vi "PhotonVision_ReadTargetData.vi"() -> ()   [LabVIEW 2019]
uses:
  <vilib>/Rock Robotics/WPI/ThirdParty/PhotonVisionLib/TypeDef/PhotonPipelineResultType.ctl
  <vilib>/Rock Robotics/WPI/ThirdParty/PhotonVisionLib/TypeDef/PhotonTrackedTargetType.ctl
  <vilib>/Rock Robotics/WPI/ThirdParty/PhotonVisionLib/TypeDef/TargetCornerType.ctl
  <vilib>/Rock Robotics/WPI/ThirdParty/JAS_Junk/TrajLib/TypeDef/TRANSFORM3D.ctl
  <vilib>/Rock Robotics/WPI/ThirdParty/JAS_Junk/TrajLib/TypeDef/TRANSLATION3D.ctl
  <vilib>/Rock Robotics/WPI/ThirdParty/JAS_Junk/TrajLib/TypeDef/ROTATION3D.ctl
  <vilib>/Rock Robotics/WPI/ThirdParty/JAS_Junk/TrajLib/TypeDef/QUATERNION.ctl
  <vilib>/Rock Robotics/WPI/ThirdParty/PhotonVisionLib/TypeDef/PhotonMultiTargetPNPResultType.ctl
  <vilib>/Rock Robotics/WPI/ThirdParty/PhotonVisionLib/TypeDef/PhotonPNPResultType.ctl
  <vilib>/Rock Robotics/WPI/ThirdParty/PhotonVisionLib/TypeDef/PhotonPipelineMetadataType.ctl
  <vilib>/Rock Robotics/WPI/ThirdParty/PhotonVisionLib/SubVI/PhotonPipelineResult_Unpack.vi
  <vilib>/Rock Robotics/WPI/ThirdParty/PhotonVisionLib/SubVI/PhotonPipelineResult_GetTargetCount.vi
  <vilib>/Rock Robotics/WPI/ThirdParty/PhotonVisionLib/SubVI/PhotonPipelineResult_GetMetadata.vi
  <vilib>/Rock Robotics/WPI/ThirdParty/PhotonVisionLib/SubVI/PhotonPipelineMetadata_GetAll.vi
  <vilib>/Rock Robotics/WPI/ThirdParty/PhotonVisionLib/SubVI/Packet_decode_ByteI8.vi
  <vilib>/Rock Robotics/WPI/ThirdParty/PhotonVisionLib/SubVI/PhotonTrackedTarget_Unpack.vi
  <vilib>/Rock Robotics/WPI/ThirdParty/PhotonVisionLib/SubVI/PhotonMultiTargetPNPResult_unpack.vi
  <vilib>/Rock Robotics/WPI/ThirdParty/PhotonVisionLib/SubVI/PhotonPipelineMetadata_Unpack.vi
  <vilib>/Rock Robotics/WPI/ThirdParty/PhotonVisionLib/SubVI/PhotonPipelineResult_New.vi
  <vilib>/Rock Robotics/WPI/ThirdParty/PhotonVisionLib/SubVI/Packet_decode_Flt64.vi
  <vilib>/Rock Robotics/WPI/ThirdParty/PhotonVisionLib/SubVI/TargetCorner_New.vi
  <vilib>/Rock Robotics/WPI/ThirdParty/PhotonVisionLib/SubVI/Packet_decode_Int32.vi
  <vilib>/Rock Robotics/WPI/ThirdParty/PhotonVisionLib/SubVI/Packet_decode_Transform3d.vi
  <vilib>/Rock Robotics/WPI/ThirdParty/PhotonVisionLib/SubVI/Packet_decode_Flt32.vi
  <vilib>/Rock Robotics/WPI/ThirdParty/PhotonVisionLib/SubVI/Packet_decode_TargetCornerArray.vi
  <vilib>/Rock Robotics/WPI/ThirdParty/PhotonVisionLib/SubVI/Packet_decode_Boolean.vi
  <vilib>/Rock Robotics/WPI/ThirdParty/PhotonVisionLib/SubVI/PhotonPNPResult_unpack.vi
  <vilib>/Rock Robotics/WPI/ThirdParty/PhotonVisionLib/SubVI/PhotonMultiTargetPNPResult_New.vi
  <vilib>/Rock Robotics/WPI/ThirdParty/PhotonVisionLib/SubVI/Packet_decode_Int16.vi
  <vilib>/Rock Robotics/WPI/ThirdParty/PhotonVisionLib/SubVI/Packet_decode_Int64.vi
  <vilib>/Rock Robotics/WPI/ThirdParty/JAS_Junk/TrajLib/VI/Transform3d_Create_Trans3dRot3d.vi
  <vilib>/Rock Robotics/WPI/ThirdParty/JAS_Junk/TrajLib/VI/Translation3d_Create.vi
  <vilib>/Rock Robotics/WPI/ThirdParty/JAS_Junk/TrajLib/VI/Rotation3d_Create_Quaternion.vi
  <vilib>/Rock Robotics/WPI/ThirdParty/JAS_Junk/TrajLib/VI/Quaternion_New.vi
  <vilib>/Rock Robotics/WPI/ThirdParty/PhotonVisionLib/SubVI/PhotonPNPResult_New.vi
  <vilib>/Rock Robotics/WPI/ThirdParty/JAS_Junk/TrajLib/VI/Quaternion_Normalize.vi
  <vilib>/Rock Robotics/WPI/ThirdParty/JAS_Junk/TrajLib/VI/Quaternion_New_Default.vi
  <vilib>/Rock Robotics/Network Tables/NT Write Boolean.vi
  <vilib>/Rock Robotics/Network Tables/NT Read Value.vi
  <vilib>/Rock Robotics/Network Tables/NT Read Raw.vi
  <vilib>/Rock Robotics/Network Tables/NT Write Number.vi
  <vilib>/Rock Robotics/WPI/ThirdParty/PhotonVisionLib/PhotonVisionLib.lvlib
  <vilib>/Rock Robotics/WPI/ThirdParty/JAS_Junk/TrajLib/Trajectory_Library.lvlib
panel:
  out "New Data":bool
  out "IsConnected":bool
  out "Has Targets":bool
  in  "CameraName":string="Microsoft LifeCam HD-3000"
  out "CtrlLibDistToBestTarg\nMeters":dbl
  out "Loop Count":i32
  out "SpecificPhotonTrackedTarget":T1={"Yaw"=0.0, "Pitch"=0.0, "Area"=0.0, "Skew"=0.0, "MinAreaRectCorners"=[], "BestCameraToTarget"={"TRANSLATION3D"={"X"=0.0, "Y"=0.0, "Z"=0.0}, "ROTATION3D"={"Q_quaternion"={"R"=1.0, "V"=[0.0, 0.0, 0.0]}}, "XF"=FALSE}, "FiducialId"=0, "AltCameraToTarget"={"TRANSLATION3D"={"X"=0.0, "Y"=0.0, "Z"=0.0}, "ROTATION3D"={"Q_quaternion"={"R"=0.0, "V"=[0.0, 0.0, 0.0]}}, "XF"=FALSE}, "PoseAmbiguity"=0.0, "DetectedCorners"=[], "ObjDetectId"=0, "ObjDetectConf"=0.0} {"AltCameraToTarget"."TRANSLATION3D"."Z" format="%14.3f"; "AltCameraToTarget"."TRANSLATION3D"."Y" format="%14.3f"; "AltCameraToTarget"."TRANSLATION3D"."X" format="%14.3f"; "BestCameraToTarget"."TRANSLATION3D"."Z" format="%14.3f"; "BestCameraToTarget"."TRANSLATION3D"."Y" format="%14.3f"; "BestCameraToTarget"."TRANSLATION3D"."X" format="%14.3f"}
  out "PipelineResult":T7={"Targets"=[], "PhotonMultiTargetPNPResult"={"PhotonPNPResult"={"IsPresent"=FALSE, "bestReprojErr"=0.0, "altReprojErr"=0.0, "ambiguity"=0.0, "Best"={"TRANSLATION3D"={"X"=0.0, "Y"=0.0, "Z"=0.0}, "ROTATION3D"={"Q_quaternion"={"R"=1.0, "V"=[0.0, 0.0, 0.0]}}, "XF"=FALSE}, "Alt"={"TRANSLATION3D"={"X"=0.0, "Y"=0.0, "Z"=0.0}, "ROTATION3D"={"Q_quaternion"={"R"=1.0, "V"=[0.0, 0.0, 0.0]}}, "XF"=FALSE}}, "FiducialIDsUsed"=[]}, "PhotonPipelineMetadata"={"CaptureTimestampMicros"=0, "PublishTimestampMicros"=0, "SequenceID"=0, "TimeSinceLastPong"=0}} {"PhotonMultiTargetPNPResult"."PhotonPNPResult"."Alt"."TRANSLATION3D"."Z" format="%14.3f"; "PhotonMultiTargetPNPResult"."PhotonPNPResult"."Alt"."TRANSLATION3D"."Y" format="%14.3f"; "PhotonMultiTargetPNPResult"."PhotonPNPResult"."Alt"."TRANSLATION3D"."X" format="%14.3f"; "PhotonMultiTargetPNPResult"."PhotonPNPResult"."Best"."TRANSLATION3D"."Z" format="%14.3f"; "PhotonMultiTargetPNPResult"."PhotonPNPResult"."Best"."TRANSLATION3D"."Y" format="%14.3f"; "PhotonMultiTargetPNPResult"."PhotonPNPResult"."Best"."TRANSLATION3D"."X" format="%14.3f"; "Targets"."AltCameraToTarget"."TRANSLATION3D"."Z" format="%14.3f"; "Targets"."AltCameraToTarget"."TRANSLATION3D"."Y" format="%14.3f"; "Targets"."AltCameraToTarget"."TRANSLATION3D"."X" format="%14.3f"; "Targets"."BestCameraToTarget"."TRANSLATION3D"."Z" format="%14.3f"; "Targets"."BestCameraToTarget"."TRANSLATION3D"."Y" format="%14.3f"; "Targets"."BestCameraToTarget"."TRANSLATION3D"."X" format="%14.3f"}
  out "SpecificTargetFound":bool
  out "TagTarget Index":i32
  in  "Fiiducial ID\n(April Tag Number)":i32
  out "BestTargetFound":bool
  out "BestYaw":dbl
  out "DistanceToBestTarget \nMeters":dbl
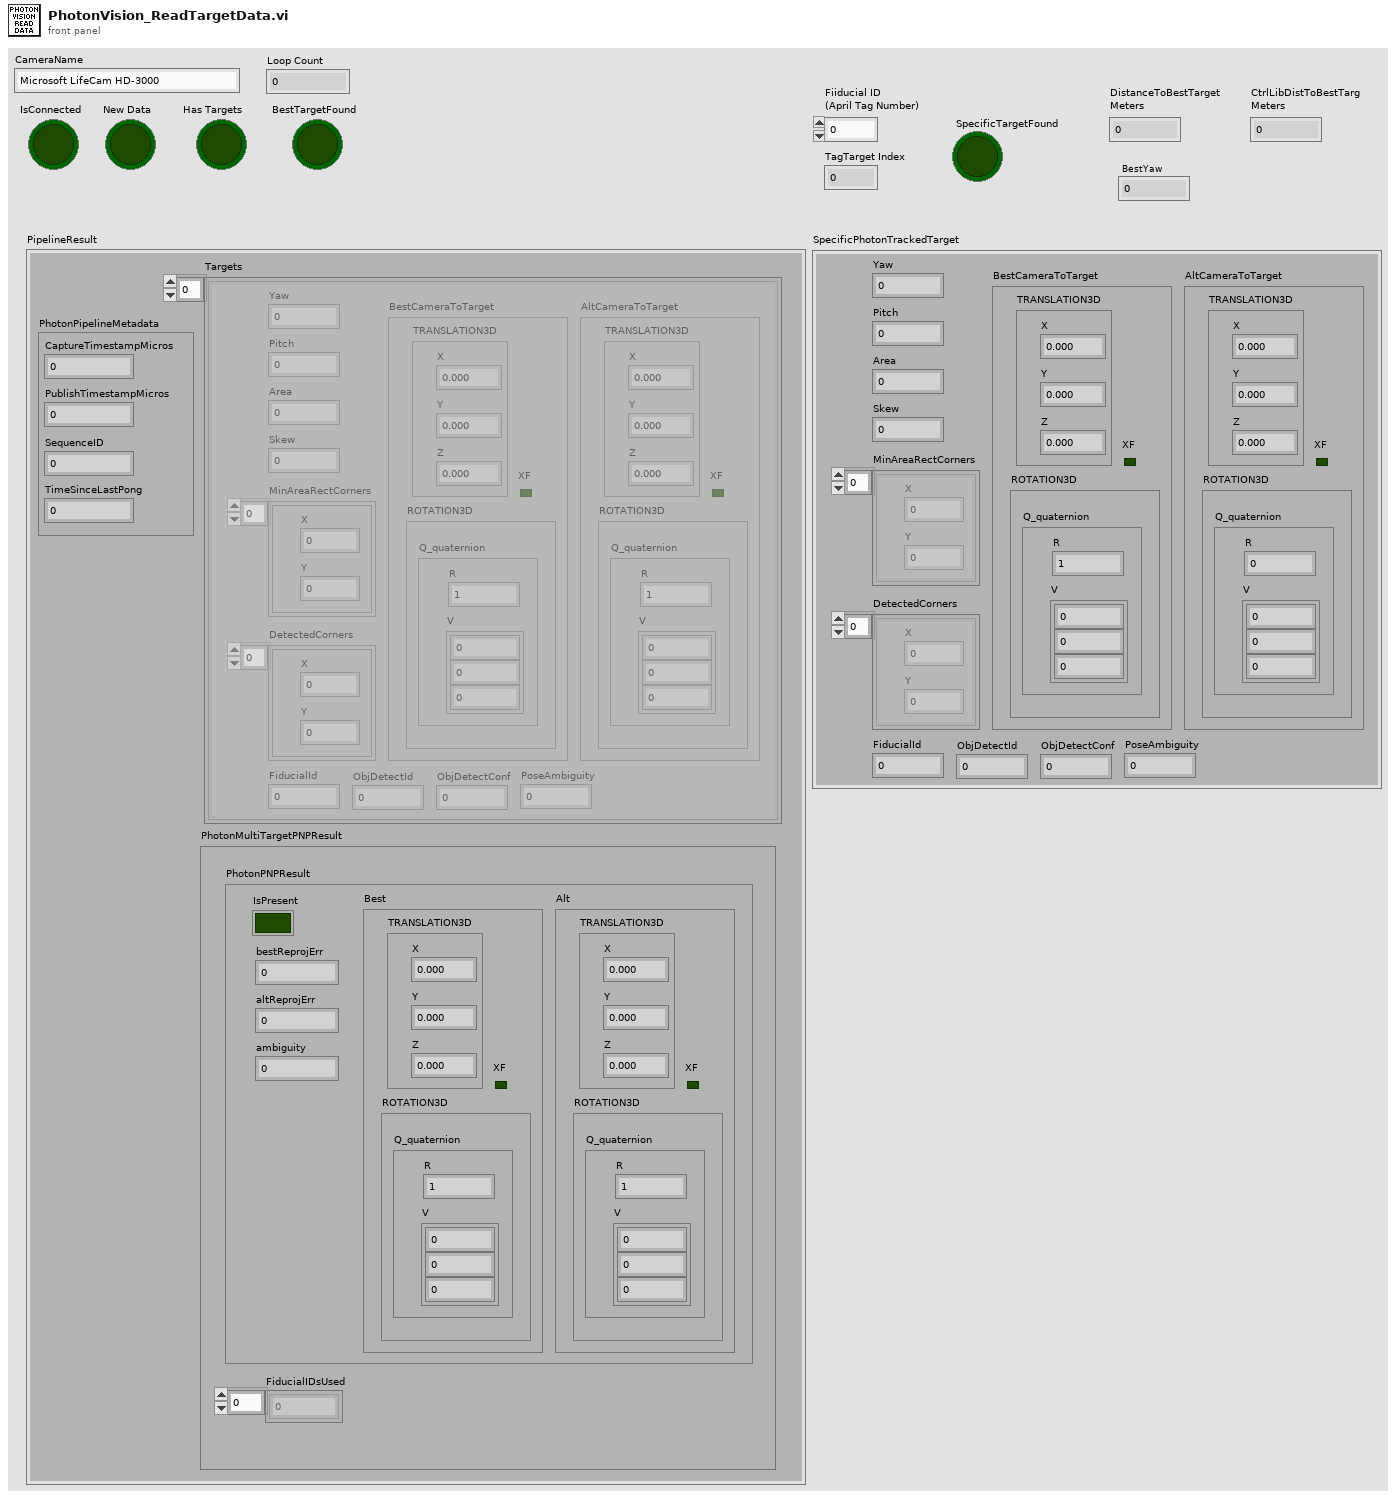
[diagram p1: front panel]
types:
  T1 = typedef "PhotonVisionLib.lvlib/PhotonTrackedTargetType.ctl" = cluster{"Yaw":dbl, "Pitch":dbl, "Area":dbl, "Skew":dbl, "MinAreaRectCorners":T2[], "BestCameraToTarget":T3, "FiducialId":i32, "AltCameraToTarget":T3, "PoseAmbiguity":dbl, "DetectedCorners":T2[], "ObjDetectId":i32, "ObjDetectConf":sgl}
  T2 = typedef "PhotonVisionLib.lvlib/TargetCornerType.ctl" = cluster{"X":dbl, "Y":dbl}
  T3 = typedef "Trajectory_Library.lvlib/TRANSFORM3D.ctl" = cluster{"TRANSLATION3D":T4, "ROTATION3D":T5, "XF":bool}
  T4 = typedef "Trajectory_Library.lvlib/TRANSLATION3D.ctl" = cluster{"X":dbl, "Y":dbl, "Z":dbl}
  T5 = typedef "Trajectory_Library.lvlib/ROTATION3D.ctl" = cluster{"Q_quaternion":T6}
  T6 = typedef "Trajectory_Library.lvlib/QUATERNION.ctl" = cluster{"R":dbl, "V":dbl[]}
  T7 = typedef "PhotonVisionLib.lvlib/PhotonPipelineResultType.ctl" = cluster{"Targets":T1[], "PhotonMultiTargetPNPResult":T8, "PhotonPipelineMetadata":T10}
  T8 = typedef "PhotonVisionLib.lvlib/PhotonMultiTargetPNPResultType.ctl" = cluster{"PhotonPNPResult":T9, "FiducialIDsUsed":i16[]}
  T9 = typedef "PhotonVisionLib.lvlib/PhotonPNPResultType.ctl" = cluster{"IsPresent":bool, "bestReprojErr":dbl, "altReprojErr":dbl, "ambiguity":dbl, "Best":T3, "Alt":T3}
  T10 = typedef "PhotonVisionLib.lvlib/PhotonPipelineMetadataType.ctl" = cluster{"CaptureTimestampMicros":i64, "PublishTimestampMicros":i64, "SequenceID":i64, "TimeSinceLastPong":i64}
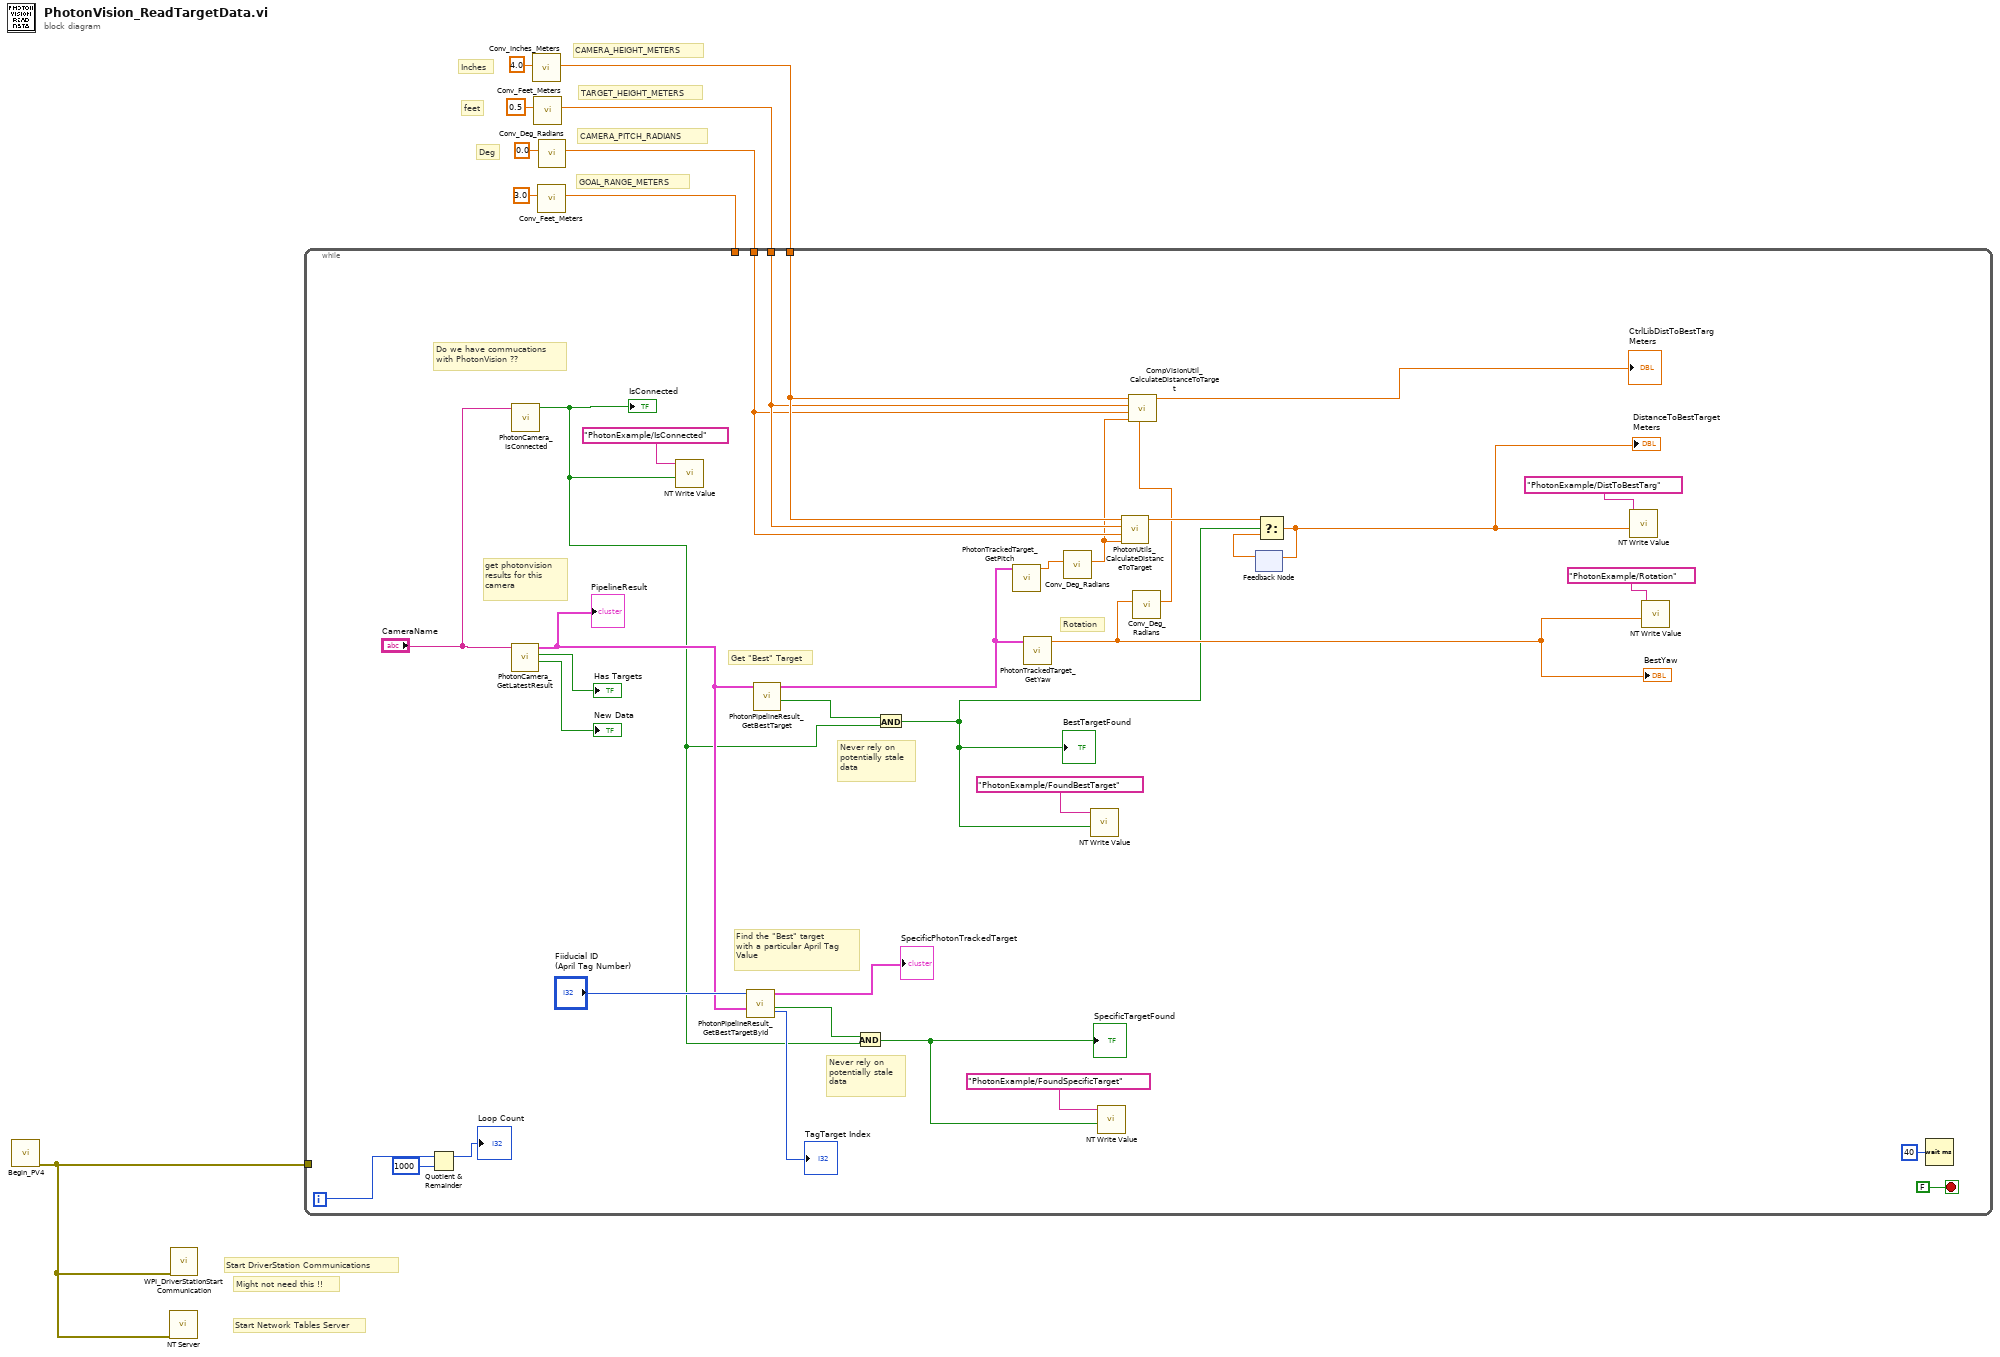
[diagram p0: block diagram]
diagram:
  # "Might not need this !!"
  # "Deg"
  # "feet"
  # "Inches"
  # "GOAL_RANGE_METERS"
  # "CAMERA_PITCH_RADIANS"
  # "TARGET_HEIGHT_METERS"
  # "CAMERA_HEIGHT_METERS"
  # "Start Network Tables Server"
  # "Start DriverStation Communications"
  n1 = call "Begin_PV4.vi"() -> ("error out"=w1:errorcluster)  [unwired: 11 in]
  n2 = call <vilib>:"NT Server.vi"("error in (no error)"=w1) -> ()  [unwired: 10 in, 1 out]
  n3 = call <vilib>:"WPI_DriverStationStart Communication.vi"("error in (no error)"=w1) -> ()  [unwired: 11 in]
  n4 = call <vilib>:"Conv_Inches_Meters.vi"("INCH"=4.0) -> ("Meters"=w5:dbl)  [unwired: 10 in]
  n5 = call <vilib>:"Conv_Feet_Meters.vi"("Feet"=0.5) -> ("Meters"=w4:dbl)  [unwired: 10 in]
  n6 = call <vilib>:"Conv_Feet_Meters.vi"("Feet"=3.0) -> ("Meters"=w2:dbl)  [unwired: 10 in]
  n7 = call <vilib>:"Conv_Deg_Radians.vi"("Degress"=0.0) -> ("Radians"=w3:dbl)  [unwired: 10 in]
  n8 = while {
    tunnel: w5 -> [w25]
    tunnel: w4 -> [w24]
    tunnel: w3 -> [w23]
    tunnel: w2 -> [_]
    tunnel: w1 -> [_]
    i -> [w28]
    stop <- FALSE stop-if-true
    # "Never rely on\npotentially stale\ndata"
    # "Never rely on\npotentially stale\ndata"
    # "Do we have commucations\nwith PhotonVision ??"
    # "Find the \"Best\" target\nwith a particular April Tag\nValue"
    # "Get \"Best\" Target"
    # "Rotation"
    # "get photonvision\nresults for this\ncamera"
    n9 = Quotient & Remainder(x=w28, y=1000) -> (x-y*floor(x/y)=→"Loop Count":i32)  [unwired: 1 out]
    n10 = call <vilib>:"PhotonCamera_GetLatestResult.vi"("CameraName"="CameraName") -> ("New Data"=→"New Data":bool, "HasTargets"=→"Has Targets":bool, "PipelineResult"=w32:T7)  [unwired: 6 in, 2 out]
    "PipelineResult" <- w32
    n11 = call <vilib>:"PhotonCamera_IsConnected.vi"("CameraName"="CameraName") -> ("IsConnected"=w12:bool)  [unwired: 9 in, 1 out]
    "IsConnected" <- w12
    n12 = call-poly <vilib>:"NT Write Value.vi"("value"=w12, "name"="PhotonExample/IsConnected" ("Name")) -> ()  [unwired: 9 in, 1 out]
    n13 = call <vilib>:"PhotonPipelineResult_GetBestTargetById.vi"("PhotonPipelineResult"=w32, "FiducialId"="Fiiducial ID\n(April Tag Number)") -> ("Target Found"=w13:bool, "PhotonTrackedTarget"=→"SpecificPhotonTrackedTarget":T1, "Target Index"=→"TagTarget Index":i32)  [unwired: 7 in]
    n14 = call <vilib>:"PhotonPipelineResult_GetBestTarget.vi"("PhotonPipelineResult"=w32) -> ("TargetFound"=w16:bool, "PhotonTrackedTarget"=w33:T1)  [unwired: 9 in]
    n15 = And(x=w13, y=w12) -> (x .and. y?=w14:bool)
    "SpecificTargetFound" <- w14
    n16 = And(x=w16, y=w12) -> (x .and. y?=w15:bool)
    "BestTargetFound" <- w15
    n17 = call <vilib>:"PhotonTrackedTarget_GetPitch.vi"("TrackedTarget"=w33) -> ("Pitch"=w35:dbl)  [unwired: 10 in]
    n18 = call <vilib>:"PhotonTrackedTarget_GetYaw.vi"("TrackedTarget"=w33) -> ("Yaw"=w21:dbl)  [unwired: 10 in]
    "BestYaw" <- w21
    n19 = call <vilib>:"Conv_Deg_Radians.vi"("Degress"=w35) -> ("Radians"=w22:dbl)  [unwired: 10 in]
    n20 = call-poly <vilib>:"NT Write Value.vi"("value"=w15, "name"="PhotonExample/FoundBestTarget" ("Name")) -> ()  [unwired: 9 in, 1 out]
    n21 = call-poly <vilib>:"NT Write Value.vi"("value"=w14, "name"="PhotonExample/FoundSpecificTarget" ("Name")) -> ()  [unwired: 9 in, 1 out]
    n22 = call <vilib>:"PhotonUtils_CalculateDistanceToTarget.vi"("TargetPitch_Radians"=w22, "CameraPitch_Radians"=w23, "TargetHeight_Meters"=w24, "CameraHeight_Meters"=w25) -> ("DistanceToTarget_Meters"=w38:dbl)  [unwired: 7 in]
    n23 = call <vilib>:"Conv_Deg_Radians.vi"("Degress"=w21) -> ("Radians"=w20:dbl)  [unwired: 10 in]
    n24 = call <vilib>:"CompVisionUtil_CalculateDistanceToTarget.vi"("TargetYawRadians"=w20, "targetPitch_Radians"=w22, "cameraPitch_Radians"=w23, "targetHeight_Meters"=w24, "cameraHeight_Meters"=w25) -> ("DistanceToTarget_Meters"=→"CtrlLibDistToBestTarg\nMeters":dbl)  [unwired: 6 in]
    n25 = feedback #1() -> (w36:dbl)  [unwired: 1 in]
    n26 = Select(t=w38, s=w15, f=w36) -> (s? t:f=w37:dbl)
    "DistanceToBestTarget \nMeters" <- w37
    n27 = feedback-in #1(w37) -> ()
    n28 = call-poly <vilib>:"NT Write Value.vi"("value"=w37, "name"="PhotonExample/DistToBestTarg" ("Name")) -> ()  [unwired: 9 in, 1 out]
    n29 = call-poly <vilib>:"NT Write Value.vi"("value"=w21, "name"="PhotonExample/Rotation" ("Name")) -> ()  [unwired: 9 in, 1 out]
    n30 = Wait (ms)(milliseconds to wait=u32 40) -> ()  [unwired: 1 out]
  }
